vi "Disconnect.vi"(8 "error in":errorcluster, 11 "34980A in":refnum<class "34980A.lvclass">) -> (0 "error out":errorcluster, 3 "34980A out":refnum<class "34980A.lvclass">)   [LabVIEW 2019, in "34980A.lvlib" / "34980A.lvclass"]
uses:
  Library/34980A.lvclass
  builds/Instruments/MLTFNC.lvlibp/Library/MLTFNC.lvclass
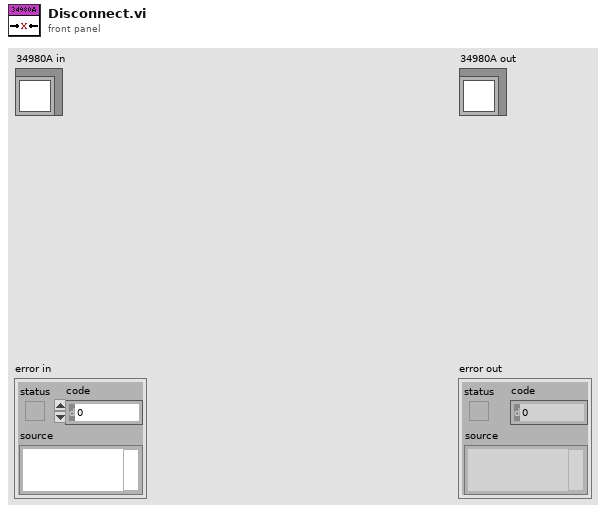
[diagram p1: front panel]
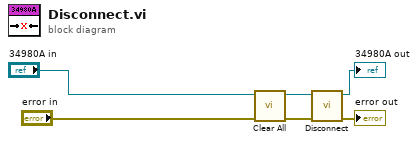
[diagram p0: block diagram]
diagram:
  n1 = call-dynamic "Clear All.vi"("error in"="error in", "34980A in"="34980A in") -> ("error out"=w1:errorcluster, "34980A out"=w2:refnum<class "34980A.lvclass">)  [unwired: 8 in]
  n2 = call-parent "Disconnect.vi"("error in"=w1, "MLTFNC in"=w2) -> ("error out"=→"error out":errorcluster, "MLTFNC out"=→"34980A out":refnum<class "34980A.lvclass">)  [unwired: 8 in]
